vi "OSICS_Set_Mode_SWT-APC.vi"(7 "OSICS slot":i32=1 min=1 max=8 step=1, 8 "error in":errorcluster, 10 "Mode":enum16{"MODE ECL", "MODE SWT"}(ring), 11 "VISA IN":refnum<visa-resource-name>) -> (0 "error out":errorcluster, 3 "VISA OUT":refnum<visa-resource-name>, 5 "ERR":i32)   [LabVIEW 2014, in "OSICS_LIB.lvlib"]
doc: "This Vi sets the operating mode of the SWT-APC (Automatic Power-Control). \nModes:\nSWT - Switch\nMODE ECL - Full-Band"
uses:
  OSICS_LIB.lvlib
panel:
  # "Basic Function to set the power units and power output\nfor the OSICS"
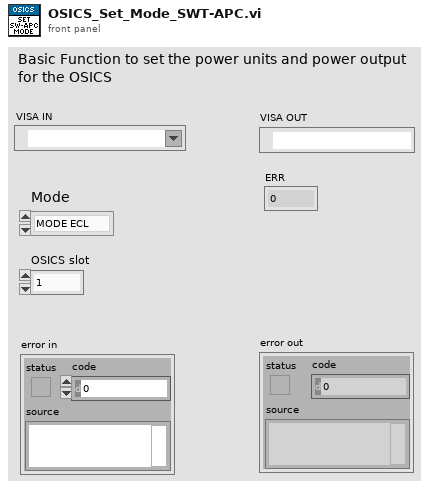
[diagram p1: front panel]
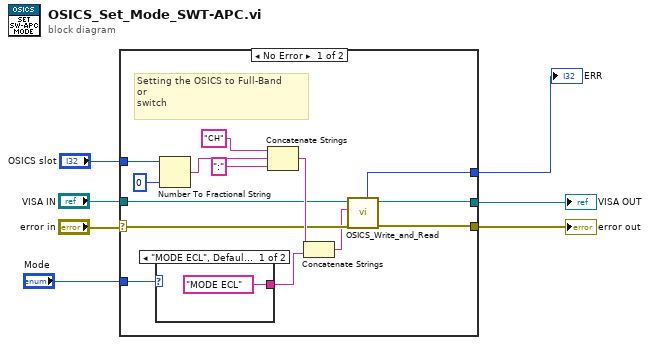
[diagram p0: block diagram]
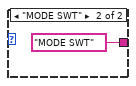
[diagram p2: hidden frame]
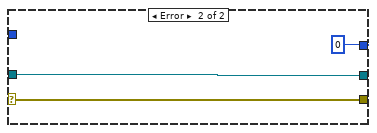
[diagram p3: hidden frame]
diagram:
  n1 = case shown="No Error" "error in" {
    selector: "error in" -> [w15 w25]
    tunnel: "VISA IN" -> [w14 w26]
    tunnel: [w10 w26] -> w6
    tunnel: [w9 w25] -> w5
    tunnel: [w12 0 ("ERR")] -> w3
    tunnel: "OSICS slot" -> [w21 _]
    tunnel: "Mode" -> [w8 _]
    frame No Error {
      # "Setting the OSICS to Full-Band\nor\nswitch"
      n2 = case shown="\"MODE ECL\", Default" w8 {
        tunnel: ["MODE ECL" ("string") "MODE SWT" ("string")] -> w11
        frame "MODE ECL", Default {
        }
        frame "MODE SWT" {
        }
      }
      n3 = Number To Fractional String(number=w21, precision (6)=i16 0) -> (F-format string=w18:string)  [unwired: 2 in]
      n4 = Concatenate Strings("CH" ("string"), w18, ":" ("string")) -> (w16:string)
      n5 = Concatenate Strings(w16, w11) -> (w13:string)
      n6 = call "OSICS_Write_and_Read.vi"("error in (no error)"=w15, "String to Send"=w13, "VISA IN"=w14) -> ("error out"=w9:errorcluster, "VISA OUT"=w10:refnum<visa-resource-name>, "ERR"=w12:i32)  [unwired: 5 in, 1 out]
    }
    frame Error {
    }
  }
  "error out" <- w5
  "VISA OUT" <- w6
  "ERR" <- w3
